vi "DANO1.vi"() -> ()   [LabVIEW 2016]
uses:
  GitHub/UCSB-Gantry/V5/Classes/Controller/Controller.lvclass
  GitHub/UCSB-Gantry/V5/Classes/Controller/Motion/Motion.lvclass
panel:
  in  "stop":bool
  in  "XYZTheta In":dbl[](array[numeric])
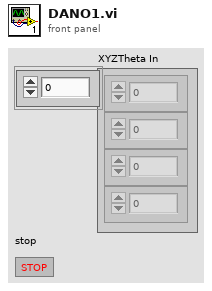
[diagram p1: front panel]
types:
  T1 = typedef "Controller.lvclass/Controllers.ctl" = cluster{"I-O.lvclass":refnum<class "I-O.lvclass">, "Motion.lvclass":refnum<class "Motion.lvclass">, "Dispenser.lvclass":refnum<class "Dispenser.lvclass">}
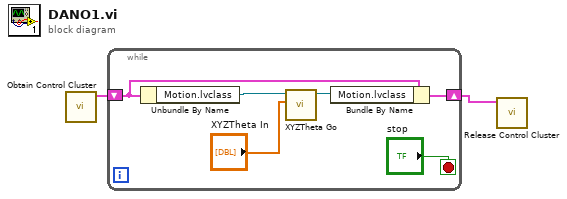
[diagram p0: block diagram]
diagram:
  n1 = call "Obtain Control Cluster.vi"() -> ("Control Out"=w2:T1)  [unwired: 11 in]
  n2 = while {
    shift-right: [w6] -> w1
    shift-left: w2 -> [w5]
    stop <- "stop" stop-if-true
    n3 = Unbundle By Name(w5) -> ("Motion.lvclass"=w8:refnum<class "Motion.lvclass">)
    n4 = call "XYZTheta Go.vi"("XYZTheta In"="XYZTheta In", "Motion in"=w8) -> ("Motion out"=w4:refnum<class "Motion.lvclass">)  [unwired: 7 in, 2 out]
    n5 = Bundle By Name(cluster=w5, "Motion.lvclass"=w4) -> (w6:T1)
  }
  n6 = call "Release Control Cluster.vi"("output cluster"=w1) -> ()  [unwired: 11 in]
